vi "AO Array Add or Remove.vi"(8 "error in (no error)":errorcluster, 10 "Size":i32, 11 "AO Channels in":T1 {"Phase" format="%.3g"; "Frequency" min=0.0001 max=10000.0 format="%.3g"; "Offset" format="%.3p"; "Amplitude" min=0.0 max=10.0 format="%.3p"}) -> (0 "error out":errorcluster, 3 "AO Channels out":T1 {"Phase" format="%.3g"; "Frequency" min=0.0001 max=10000.0 format="%.3g"; "Offset" format="%.3p"; "Amplitude" min=0.0 max=10.0 format="%.3p"})   [LabVIEW 2019, in "Instrument.Lockin.lvclass"]
uses:
  Instrument.Lockin.lvclass
  Instrument.DAQ/Typedefs/AO.Channel--Cluster--Array.ctl
  Instrument.DAQ/Typedefs/AO.Channel--Cluster.ctl
  Instrument.DAQ/Typedefs/AO.Function--Enum.ctl
  Instrument.DAQ/Instrument.DAQ.lvclass
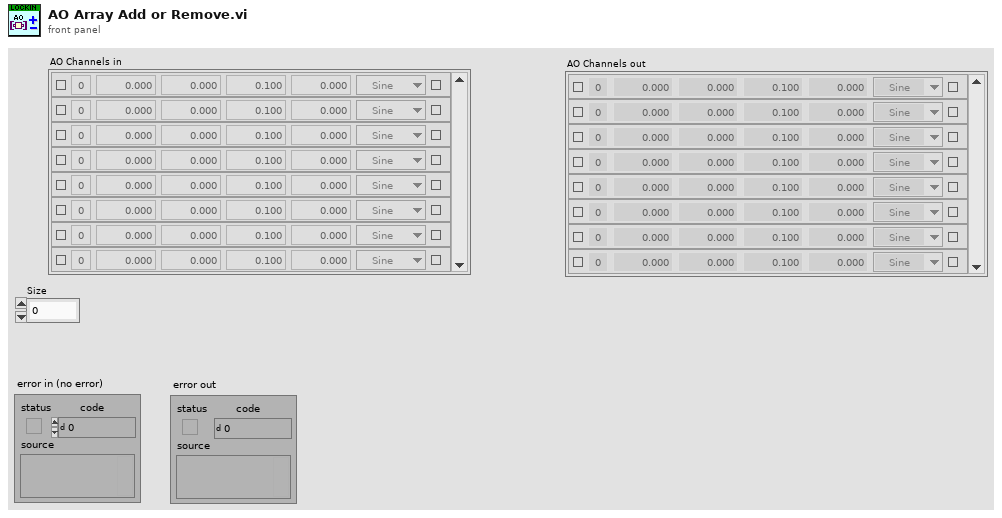
[diagram p1: front panel]
types:
  T1 = typedef "Instrument.DAQ.lvclass/AO.Channel--Cluster--Array.ctl" = T2[]
  T2 = typedef "Instrument.DAQ.lvclass/AO.Channel--Cluster.ctl" = cluster{"Enable?":bool, "Channel":i32, "Amplitude":dbl, "Offset":dbl, "Frequency":dbl, "Phase":dbl, "Function":T3, "Sweeping?":bool}
  T3 = typedef "Instrument.DAQ.lvclass/AO.Function--Enum.ctl" = enum16{"Sine", "Triangle", "Square"}
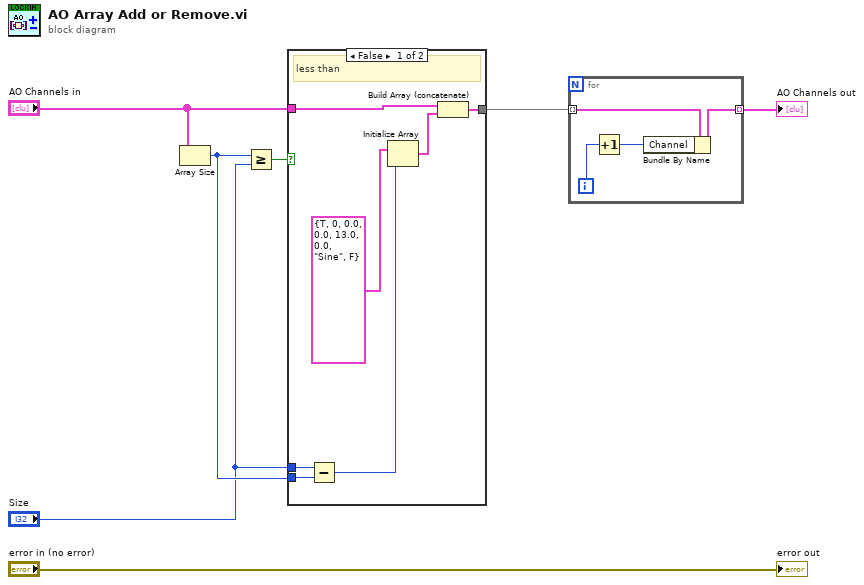
[diagram p0: block diagram]
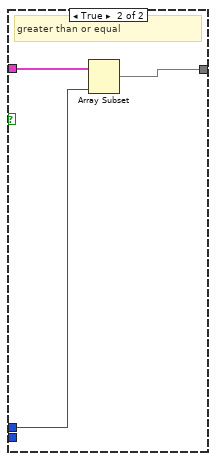
[diagram p2: hidden frame]
diagram:
  n1 = Array Size(array="AO Channels in") -> (size(s)=w7:i32)
  n2 = Greater Or Equal?(x=w7, y="Size") -> (x >= y?=w6:bool)
  n3 = case shown="False" w6 {
    tunnel: "AO Channels in" -> [w9 w17]
    tunnel: "Size" -> [w12 w16]
    tunnel: [w13 w15] -> w3
    tunnel: w7 -> [w11 _]
    frame False {
      # "less than"
      n4 = Subtract(x=w12, y=w11) -> (x-y=w10:i32)
      n5 = Initialize Array(T2 {"Enable?"=TRUE, "Channel"=0, "Amplitude"=0.0, "Offset"=0.0, "Frequency"=13.0, "Phase"=0.0, "Function"=enum."Sine", "Sweeping?"=FALSE} ("AO"), w10) -> (w14:T2[])
      n6 = Build Array (concatenate)(w9, w14) -> (w13:T1)
    }
    frame True {
      # "greater than or equal"
      n7 = Array Subset(array=w17, length=w16) -> (w15:T1)  [unwired: 1 in]
    }
  }
  n8 = for {
    tunnel: w3 -> [w21] mode=indexing
    tunnel: [w20] -> w2 mode=indexing
    i -> [w18]
    n9 = Increment(x=w18) -> (x+1=w19:i32)
    n10 = Bundle By Name(cluster=w21, "Channel"=w19) -> (w20:T2)
  }
  "AO Channels out" <- w2
  "error out" <- "error in (no error)"
